vi "InitDrivebase.vi"   [LabVIEW 2020]
doc: "This VI initializes devices related directly to the drive subsystem."
uses:
  <vilib>/Rock Robotics/WPI/Solenoid/WPI_SolenoidChannel.ctl
  <vilib>/Rock Robotics/WPI/ThirdParty/Phoenix-LabVIEW/Motor Controller/Controls/CTRE_Phoenix_MotorControl_SupplyCurrentLimitConfiguration.ctl
  <vilib>/Rock Robotics/WPI/ThirdParty/Phoenix-LabVIEW/Motor Controller/Controls/CTRE_Phoenix_MotorControl_TalonFXInvertType.ctl
  <vilib>/Rock Robotics/WPI/ThirdParty/Phoenix-LabVIEW/Motor Controller/Controls/CTRE_Phoenix_MotorControl_NeutralMode.ctl
  <vilib>/Rock Robotics/WPI/ThirdParty/Phoenix-LabVIEW/Motor Controller/Controls/CTRE_Phoenix_MotorControl_FeedbackDevice_TalonFX.ctl
  <vilib>/Rock Robotics/WPI/ThirdParty/Phoenix-LabVIEW/Motor Controller/Controls/CTRE_Phoenix_MotorControl_StatusFrameEnhanced.ctl
  <vilib>/Rock Robotics/WPI/ThirdParty/Phoenix-LabVIEW/Motor Controller/Controls/CTRE_Phoenix_MotorControl_StatorCurrentLimitConfiguration.ctl
  <vilib>/Rock Robotics/WPI/Solenoid/WPI_SolenoidOpenDouble.vi
  GlobalDrivebase.vi
types:
  T1 = typedef "CTRE_Phoenix_MotorControl_StatorCurrentLimitConfiguration.ctl" = cluster{"Enable?":bool, "Current Limit":dbl, "Threshold Current":dbl, "Threshold Time":dbl}
  T2 = typedef "CTRE_Phoenix_MotorControl_StatusFrameEnhanced.ctl" = u16
  T3 = typedef "WPI_SolenoidChannel.ctl" = enum8{"Solenoid 0", "Solenoid 1", "Solenoid 2", "Solenoid 3", "Solenoid 4", "Solenoid 5", "Solenoid 6", "Solenoid 7", "Solenoid 8", "Solenoid 9", "Solenoid 10", "Solenoid 11", "Solenoid 12", "Solenoid 13", "Solenoid 14", "Solenoid 15", "Invalid"}
  T4 = typedef "CTRE_Phoenix_MotorControl_TalonFXInvertType.ctl" = enum16{"Counter-Clockwise", "Clockwise"}
  T5 = typedef "CTRE_Phoenix_MotorControl_FeedbackDevice_TalonFX.ctl" = i8
  T6 = typedef "CTRE_Phoenix_MotorControl_SupplyCurrentLimitConfiguration.ctl" = cluster{"Enable?":bool, "Current Limit":dbl, "Threshold Current":dbl, "Threshold Time":dbl}
  T7 = typedef "CTRE_Phoenix_MotorControl_NeutralMode.ctl" = enum8{"EEPROMSetting", "Override to Coast", "Override to Brake"}
  T8 = typedef "CTRE_PigeonIMU_DeviceRef.ctl" = cluster{"DeviceStatus":errorcluster, "Device Number":u8, "Type":T9, "Device ID":u32, "Handle":u64, "UsageFrame":u32, "Library Path":path}
  T9 = typedef "CTRE_PigeonIMU_ConnectionType.ctl" = u32
  T10 = typedef "WPI_MotorControlDeviceRef.ctl" = cluster{"DeviceStatus":errorcluster, "Type":T11, "PWM":cluster{"PWM Channel":T12, "DeadBand":T13}, "CAN":cluster{"Device Number":u8, "SetOutput VI Ref":variant, "GetOutput VI Ref":variant, "Enable VI Ref":variant, "Disable VI Ref":variant, "Data":variant}, "Invert":bool, "DIO PWM":cluster{"PWM \"Enable\" Channel":T12, "DIOChannel":T14, "PWM Rate":dbl}}
  T11 = typedef "WPI_MotorControlType.ctl" = enum16{"PWM", "CAN", "DIO PWM"}
  T12 = typedef "FPGA_DIOPWMChannel.ctl" = enum8{"PWM 0", "PWM 1", "PWM 2", "PWM 3", "PWM 4", "PWM 5", "PWM 6", "PWM 7", "PWM 8", "PWM 9", "PWM MXP 0", "PWM MXP 1", "PWM MXP 2", "PWM MXP 3", "PWM MXP 4", "PWM MXP 5", "PWM MXP 6", "PWM MXP 7", "PWM MXP 8", "PWM MXP 9", "Invalid"}
  T13 = typedef "WPI_PWMDeadband.ctl" = cluster{"Name":string, "maxPositivePwm":i32, "minPositivePwm":i32, "centerPwm":i32, "maxNegativePwm":i32, "minNegativePwm":i32, "angularRange":u16}
  T14 = typedef "FPGA_DIOChannel.ctl" = enum8{"DIO 0", "DIO 1", "DIO 2", "DIO 3", "DIO 4", "DIO 5", "DIO 6", "DIO 7", "DIO 8", "DIO 9", "DIO MXP 0", "DIO MXP 1", "DIO MXP 2", "DIO MXP 3", "DIO MXP 4", "DIO MXP 5", "DIO MXP 6", "DIO MXP 7", "DIO MXP 8", "DIO MXP 9", "DIO MXP 10", "DIO MXP 11", "DIO MXP 12", "DIO MXP 13", "DIO MXP 14", "DIO MXP 15", "SPI Port CS1", "SPI Port CS2", "SPI Port CS3", "SPI Port MISO", "SPI Port MOSI", "Invalid"}
  T15 = typedef "WPI_SolenoidDevRef.ctl" = cluster{"DevStatus":errorcluster, "Pneumatics Control Module":u8, "Forward Solenoid Channel":T3, "Reverse Solenoid Channel":T3}
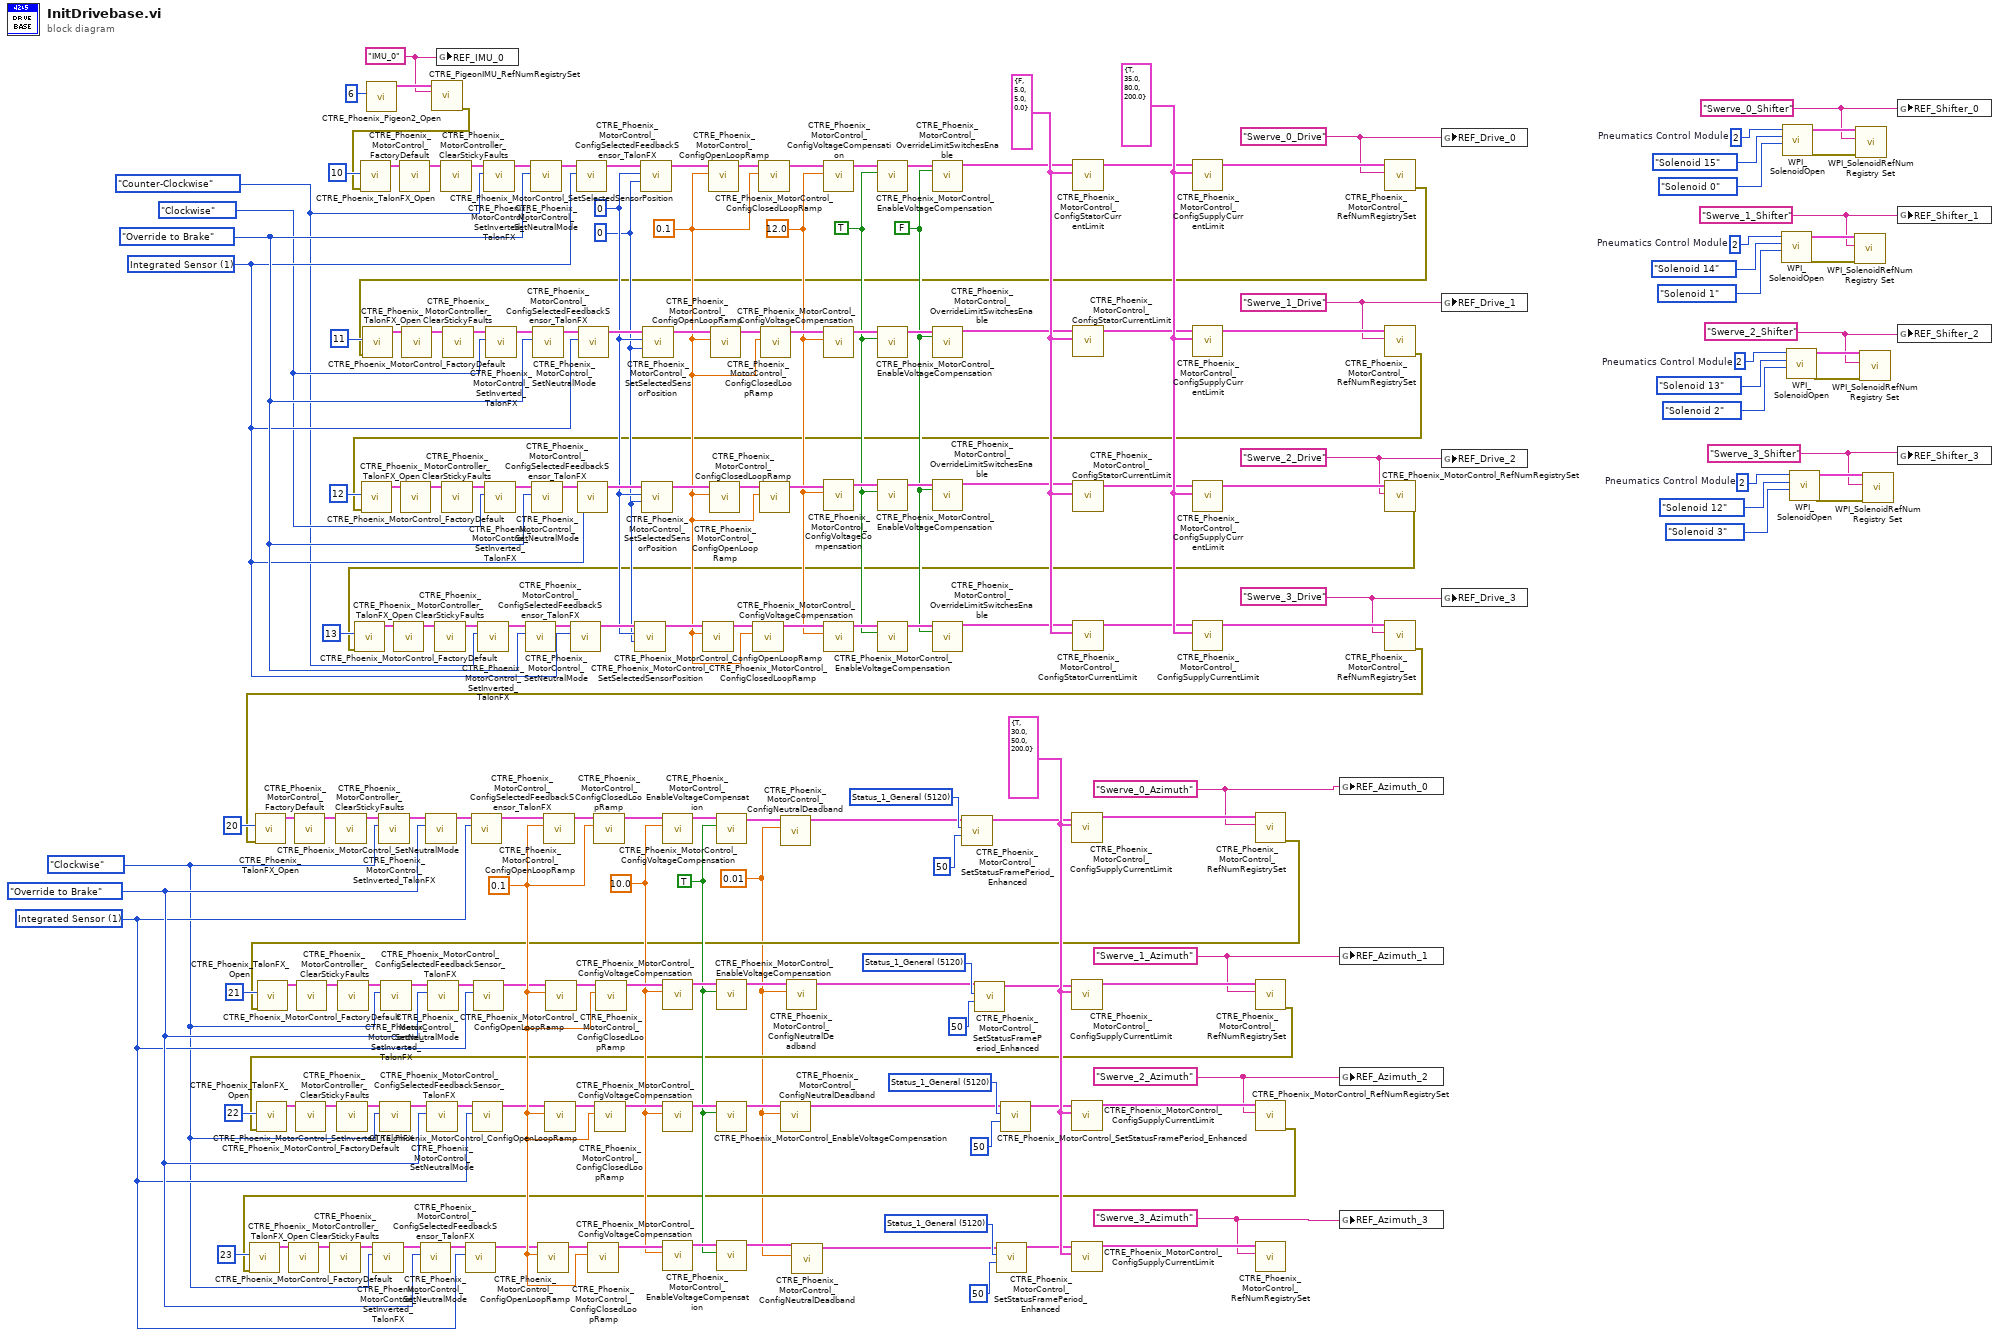
[diagram p0: block diagram]
diagram:
  w1 = "IMU_0" ("refnum name")
  w21 = 0.01 ("Percent Deadband")
  w34 = T1 {"Enable?"=FALSE, "Current Limit"=5.0, "Threshold Current"=5.0, "Threshold Time"=0.0} ("Stator Current Limit Configuration")
  w40 = T2 5120 items=["Status_1_General"=5120, "Status_2_Feedback0"=5184, "Status_3_Quadrature"=5248, "Status_4_AinTempVbat"=5312, "Status_6_Misc"=5440, "Status_7_CommStatus"=5504, "Status_8_PulseWidth"=5568, "Status_9_MotProfBuffer"=5632, "Status_10_MotionMagic"=5696, "Status_11_UartGadgeteer"=5760, "Status_12_Feedback1"=5824, "Status_13_Base_PIDF0"=5888, "Status_14_Turn_PIDF1"=5952, "Status_15_FirmwareApiStatus"=6016, "Status_Brushless_Current"=4672] ("Status Frame")
  w43 = T2 5120 items=["Status_1_General"=5120, "Status_2_Feedback0"=5184, "Status_3_Quadrature"=5248, "Status_4_AinTempVbat"=5312, "Status_6_Misc"=5440, "Status_7_CommStatus"=5504, "Status_8_PulseWidth"=5568, "Status_9_MotProfBuffer"=5632, "Status_10_MotionMagic"=5696, "Status_11_UartGadgeteer"=5760, "Status_12_Feedback1"=5824, "Status_13_Base_PIDF0"=5888, "Status_14_Turn_PIDF1"=5952, "Status_15_FirmwareApiStatus"=6016, "Status_Brushless_Current"=4672] ("Status Frame")
  w46 = T2 5120 items=["Status_1_General"=5120, "Status_2_Feedback0"=5184, "Status_3_Quadrature"=5248, "Status_4_AinTempVbat"=5312, "Status_6_Misc"=5440, "Status_7_CommStatus"=5504, "Status_8_PulseWidth"=5568, "Status_9_MotProfBuffer"=5632, "Status_10_MotionMagic"=5696, "Status_11_UartGadgeteer"=5760, "Status_12_Feedback1"=5824, "Status_13_Base_PIDF0"=5888, "Status_14_Turn_PIDF1"=5952, "Status_15_FirmwareApiStatus"=6016, "Status_Brushless_Current"=4672] ("Status Frame")
  w48 = T2 5120 items=["Status_1_General"=5120, "Status_2_Feedback0"=5184, "Status_3_Quadrature"=5248, "Status_4_AinTempVbat"=5312, "Status_6_Misc"=5440, "Status_7_CommStatus"=5504, "Status_8_PulseWidth"=5568, "Status_9_MotProfBuffer"=5632, "Status_10_MotionMagic"=5696, "Status_11_UartGadgeteer"=5760, "Status_12_Feedback1"=5824, "Status_13_Base_PIDF0"=5888, "Status_14_Turn_PIDF1"=5952, "Status_15_FirmwareApiStatus"=6016, "Status_Brushless_Current"=4672] ("Status Frame")
  w58 = FALSE ("Override Limit Switch Enable?")
  w13 = "Swerve_0_Shifter" ("refnum name")
  w68 = u8 2  # Pneumatics Control Module
  w12 = "Swerve_1_Shifter" ("refnum name")
  w73 = u8 2  # Pneumatics Control Module
  w11 = "Swerve_2_Shifter" ("refnum name")
  w78 = u8 2  # Pneumatics Control Module
  w79 = CTRE_Phoenix_MotorControl_TalonFXInvertType."Counter-Clockwise" ("Invert Type")
  w81 = TRUE ("Enable Voltage Compensation?")
  w82 = 10.0 ("Saturation Voltage")
  w83 = TRUE ("Enable Voltage Compensation?")
  w84 = 12.0 ("Saturation Voltage")
  w101 = T5 1 items=["Integrated Sensor"=1, "Sensor Sum (S0 + S1)"=9, "Sensor Difference (D0 - D1)"=10, "Remote Source 0"=11, "Remote Source 1"=12, "None"=14, "Software Emulated"=15] ("Talon FX Feedback Device")
  w104 = T6 {"Enable?"=TRUE, "Current Limit"=30.0, "Threshold Current"=50.0, "Threshold Time"=200.0} ("Supply Current Limit Configuration")
  w102 = 0.1 ("secondsFromNeutralToFull")
  w103 = CTRE_Phoenix_MotorControl_NeutralMode."Override to Brake" ("Motor Control Neutral Mode")
  w63 = CTRE_Phoenix_MotorControl_TalonFXInvertType."Clockwise" ("Invert Type")
  w5 = "Swerve_0_Azimuth" ("refnum name")
  w4 = "Swerve_1_Azimuth" ("refnum name")
  w3 = "Swerve_2_Azimuth" ("refnum name")
  w2 = "Swerve_3_Azimuth" ("refnum name")
  w140 = T5 1 items=["Integrated Sensor"=1, "Sensor Sum (S0 + S1)"=9, "Sensor Difference (D0 - D1)"=10, "Remote Source 0"=11, "Remote Source 1"=12, "None"=14, "Software Emulated"=15] ("Talon FX Feedback Device")
  w142 = T6 {"Enable?"=TRUE, "Current Limit"=35.0, "Threshold Current"=80.0, "Threshold Time"=200.0} ("Supply Current Limit Configuration")
  w137 = 0.1 ("secondsFromNeutralToFull")
  w138 = u32 0 ("pidLoopIdx")
  w139 = 0 ("New Sensor Position")
  w141 = CTRE_Phoenix_MotorControl_NeutralMode."Override to Brake" ("Motor Control Neutral Mode")
  w80 = CTRE_Phoenix_MotorControl_TalonFXInvertType."Clockwise" ("Invert Type")
  w9 = "Swerve_0_Drive" ("refnum name")
  w8 = "Swerve_1_Drive" ("refnum name")
  w7 = "Swerve_2_Drive" ("refnum name")
  w6 = "Swerve_3_Drive" ("refnum name")
  w10 = "Swerve_3_Shifter" ("refnum name")
  w187 = u8 2  # Pneumatics Control Module
  n1 = call <vilib>:"CTRE_Phoenix_Pigeon2_Open.vi"("Device Number"=u8 6) -> ("PigeonIMUDevRef"=w19:T8)  [unwired: 9 in, 1 out]
  n2 = call <vilib>:"CTRE_PigeonIMU_RefNumRegistrySet.vi"("refnum name"=w1, "PigeonIMUDevRef"=w19) -> ("error out"=w15:errorcluster)  [unwired: 8 in, 1 out]
  n3 = call <vilib>:"CTRE_Phoenix_TalonFX_Open.vi"("error in"=w15, "Device Number"=u8 10 ("Drive 4L")) -> ("PhoenixMotorControlDevRef"=w148:T10)  [unwired: 8 in, 1 out]
  n4 = call <vilib>:"CTRE_Phoenix_MotorControl_FactoryDefault.vi"("PhoenixMotorControlDevRef"=w148) -> ("PhoenixMotorControlDevRef"=w146:T10)  [unwired: 9 in, 1 out]
  n5 = global write "GlobalDrivebase.vi" "REF_IMU_0"(w1) -> ()
  n6 = call <vilib>:"CTRE_Phoenix_MotorController_ClearStickyFaults.vi"("PhoenixMotorControlDevRef"=w146) -> ("PhoenixMotorControlDevRef"=w145:T10)  [unwired: 9 in, 1 out]
  n7 = call <vilib>:"CTRE_Phoenix_MotorControl_SetInverted_TalonFX.vi"("Invert Type"=w79, "PhoenixMotorControlDevRef"=w145) -> ("PhoenixMotorControlDevRef"=w152:T10)  [unwired: 8 in, 1 out]
  n8 = call <vilib>:"CTRE_Phoenix_MotorControl_SetNeutralMode.vi"("Motor Control Neutral Mode"=w141, "PhoenixMotorControlDevRef"=w152) -> ("PhoenixMotorControlDevRef"=w144:T10)  [unwired: 8 in, 1 out]
  n9 = call <vilib>:"CTRE_Phoenix_MotorControl_ConfigSelectedFeedbackSensor_TalonFX.vi"("Talon FX Feedback Device"=w140, "PhoenixMotorControlDevRef"=w144) -> ("PhoenixMotorControlDevRef"=w143:T10)  [unwired: 8 in, 1 out]
  n10 = call <vilib>:"CTRE_Phoenix_MotorControl_SetSelectedSensorPosition.vi"("pidLoopIdx"=w138, "New Sensor Position"=w139, "PhoenixMotorControlDevRef"=w143) -> ("PhoenixMotorControlDevRef"=w151:T10)  [unwired: 7 in, 1 out]
  n11 = call <vilib>:"CTRE_Phoenix_MotorControl_ConfigOpenLoopRamp.vi"("secondsFromNeutralToFull"=w137, "PhoenixMotorControlDevRef"=w151) -> ("PhoenixMotorControlDevRef"=w147:T10)  [unwired: 8 in, 1 out]
  n12 = call <vilib>:"CTRE_Phoenix_MotorControl_ConfigClosedLoopRamp.vi"("secondsFromNeutralToFull"=w137, "PhoenixMotorControlDevRef"=w147) -> ("PhoenixMotorControlDevRef"=w92:T10)  [unwired: 8 in, 1 out]
  n13 = call <vilib>:"CTRE_Phoenix_MotorControl_ConfigVoltageCompensation.vi"("Saturation Voltage"=w84, "PhoenixMotorControlDevRef"=w92) -> ("PhoenixMotorControlDevRef"=w100:T10)  [unwired: 8 in, 1 out]
  n14 = call <vilib>:"CTRE_Phoenix_MotorControl_EnableVoltageCompensation.vi"("Enable Voltage Compensation?"=w83, "PhoenixMotorControlDevRef"=w100) -> ("PhoenixMotorControlDevRef"=w62:T10)  [unwired: 8 in, 1 out]
  n15 = call <vilib>:"CTRE_Phoenix_MotorControl_OverrideLimitSwitchesEnable.vi"("PhoenixMotorControlDevRef"=w62, "Override Limit Switch Enable?"=w58) -> ("PhoenixMotorControlDevRef"=w33:T10)  [unwired: 12 in, 1 out]
  n16 = call <vilib>:"CTRE_Phoenix_MotorControl_ConfigStatorCurrentLimit.vi"("Stator Current Limit Configuration"=w34, "PhoenixMotorControlDevRef"=w33) -> ("PhoenixMotorControlDevRef"=w38:T10)  [unwired: 8 in, 1 out]
  n17 = call <vilib>:"CTRE_Phoenix_MotorControl_ConfigSupplyCurrentLimit.vi"("Supply Current Limit Configuration"=w142, "PhoenixMotorControlDevRef"=w38) -> ("PhoenixMotorControlDevRef"=w150:T10)  [unwired: 8 in, 1 out]
  n18 = global write "GlobalDrivebase.vi" "REF_Azimuth_0"(w5) -> ()
  n19 = global write "GlobalDrivebase.vi" "REF_Azimuth_1"(w4) -> ()
  n20 = global write "GlobalDrivebase.vi" "REF_Azimuth_2"(w3) -> ()
  n21 = global write "GlobalDrivebase.vi" "REF_Azimuth_3"(w2) -> ()
  n22 = call <vilib>:"CTRE_Phoenix_MotorControl_RefNumRegistrySet.vi"("refnum name"=w9, "PhoenixMotorControlDevRef"=w150) -> ("error out"=w18:errorcluster)  [unwired: 8 in, 1 out]
  n23 = call <vilib>:"CTRE_Phoenix_TalonFX_Open.vi"("error in"=w18, "Device Number"=u8 11 ("Drive 4L")) -> ("PhoenixMotorControlDevRef"=w158:T10)  [unwired: 8 in, 1 out]
  n24 = call <vilib>:"CTRE_Phoenix_MotorControl_FactoryDefault.vi"("PhoenixMotorControlDevRef"=w158) -> ("PhoenixMotorControlDevRef"=w156:T10)  [unwired: 9 in, 1 out]
  n25 = call <vilib>:"CTRE_Phoenix_MotorController_ClearStickyFaults.vi"("PhoenixMotorControlDevRef"=w156) -> ("PhoenixMotorControlDevRef"=w155:T10)  [unwired: 9 in, 1 out]
  n26 = call <vilib>:"CTRE_Phoenix_MotorControl_SetInverted_TalonFX.vi"("Invert Type"=w80, "PhoenixMotorControlDevRef"=w155) -> ("PhoenixMotorControlDevRef"=w162:T10)  [unwired: 8 in, 1 out]
  n27 = call <vilib>:"CTRE_Phoenix_MotorControl_SetNeutralMode.vi"("Motor Control Neutral Mode"=w141, "PhoenixMotorControlDevRef"=w162) -> ("PhoenixMotorControlDevRef"=w154:T10)  [unwired: 8 in, 1 out]
  n28 = call <vilib>:"CTRE_Phoenix_MotorControl_ConfigSelectedFeedbackSensor_TalonFX.vi"("Talon FX Feedback Device"=w140, "PhoenixMotorControlDevRef"=w154) -> ("PhoenixMotorControlDevRef"=w153:T10)  [unwired: 8 in, 1 out]
  n29 = call <vilib>:"CTRE_Phoenix_MotorControl_SetSelectedSensorPosition.vi"("pidLoopIdx"=w138, "New Sensor Position"=w139, "PhoenixMotorControlDevRef"=w153) -> ("PhoenixMotorControlDevRef"=w161:T10)  [unwired: 7 in, 1 out]
  n30 = call <vilib>:"CTRE_Phoenix_MotorControl_ConfigOpenLoopRamp.vi"("secondsFromNeutralToFull"=w137, "PhoenixMotorControlDevRef"=w161) -> ("PhoenixMotorControlDevRef"=w157:T10)  [unwired: 8 in, 1 out]
  n31 = call <vilib>:"CTRE_Phoenix_MotorControl_ConfigClosedLoopRamp.vi"("secondsFromNeutralToFull"=w137, "PhoenixMotorControlDevRef"=w157) -> ("PhoenixMotorControlDevRef"=w91:T10)  [unwired: 8 in, 1 out]
  n32 = call <vilib>:"CTRE_Phoenix_MotorControl_ConfigVoltageCompensation.vi"("Saturation Voltage"=w84, "PhoenixMotorControlDevRef"=w91) -> ("PhoenixMotorControlDevRef"=w99:T10)  [unwired: 8 in, 1 out]
  n33 = call <vilib>:"CTRE_Phoenix_MotorControl_EnableVoltageCompensation.vi"("Enable Voltage Compensation?"=w83, "PhoenixMotorControlDevRef"=w99) -> ("PhoenixMotorControlDevRef"=w61:T10)  [unwired: 8 in, 1 out]
  n34 = call <vilib>:"CTRE_Phoenix_MotorControl_OverrideLimitSwitchesEnable.vi"("PhoenixMotorControlDevRef"=w61, "Override Limit Switch Enable?"=w58) -> ("PhoenixMotorControlDevRef"=w32:T10)  [unwired: 12 in, 1 out]
  n35 = call <vilib>:"CTRE_Phoenix_MotorControl_ConfigStatorCurrentLimit.vi"("Stator Current Limit Configuration"=w34, "PhoenixMotorControlDevRef"=w32) -> ("PhoenixMotorControlDevRef"=w37:T10)  [unwired: 8 in, 1 out]
  n36 = call <vilib>:"CTRE_Phoenix_MotorControl_ConfigSupplyCurrentLimit.vi"("Supply Current Limit Configuration"=w142, "PhoenixMotorControlDevRef"=w37) -> ("PhoenixMotorControlDevRef"=w160:T10)  [unwired: 8 in, 1 out]
  n37 = call <vilib>:"CTRE_Phoenix_MotorControl_RefNumRegistrySet.vi"("refnum name"=w8, "PhoenixMotorControlDevRef"=w160) -> ("error out"=w17:errorcluster)  [unwired: 8 in, 1 out]
  n38 = call <vilib>:"CTRE_Phoenix_TalonFX_Open.vi"("error in"=w17, "Device Number"=u8 12 ("Drive 4L")) -> ("PhoenixMotorControlDevRef"=w168:T10)  [unwired: 8 in, 1 out]
  n39 = call <vilib>:"CTRE_Phoenix_MotorControl_FactoryDefault.vi"("PhoenixMotorControlDevRef"=w168) -> ("PhoenixMotorControlDevRef"=w166:T10)  [unwired: 9 in, 1 out]
  n40 = call <vilib>:"CTRE_Phoenix_MotorController_ClearStickyFaults.vi"("PhoenixMotorControlDevRef"=w166) -> ("PhoenixMotorControlDevRef"=w165:T10)  [unwired: 9 in, 1 out]
  n41 = call <vilib>:"CTRE_Phoenix_MotorControl_SetInverted_TalonFX.vi"("Invert Type"=w80, "PhoenixMotorControlDevRef"=w165) -> ("PhoenixMotorControlDevRef"=w172:T10)  [unwired: 8 in, 1 out]
  n42 = call <vilib>:"CTRE_Phoenix_MotorControl_SetNeutralMode.vi"("Motor Control Neutral Mode"=w141, "PhoenixMotorControlDevRef"=w172) -> ("PhoenixMotorControlDevRef"=w164:T10)  [unwired: 8 in, 1 out]
  n43 = call <vilib>:"CTRE_Phoenix_MotorControl_ConfigSelectedFeedbackSensor_TalonFX.vi"("Talon FX Feedback Device"=w140, "PhoenixMotorControlDevRef"=w164) -> ("PhoenixMotorControlDevRef"=w163:T10)  [unwired: 8 in, 1 out]
  n44 = call <vilib>:"CTRE_Phoenix_MotorControl_SetSelectedSensorPosition.vi"("pidLoopIdx"=w138, "New Sensor Position"=w139, "PhoenixMotorControlDevRef"=w163) -> ("PhoenixMotorControlDevRef"=w171:T10)  [unwired: 7 in, 1 out]
  n45 = call <vilib>:"CTRE_Phoenix_MotorControl_ConfigOpenLoopRamp.vi"("secondsFromNeutralToFull"=w137, "PhoenixMotorControlDevRef"=w171) -> ("PhoenixMotorControlDevRef"=w167:T10)  [unwired: 8 in, 1 out]
  n46 = call <vilib>:"CTRE_Phoenix_MotorControl_ConfigClosedLoopRamp.vi"("secondsFromNeutralToFull"=w137, "PhoenixMotorControlDevRef"=w167) -> ("PhoenixMotorControlDevRef"=w90:T10)  [unwired: 8 in, 1 out]
  n47 = call <vilib>:"CTRE_Phoenix_MotorControl_ConfigVoltageCompensation.vi"("Saturation Voltage"=w84, "PhoenixMotorControlDevRef"=w90) -> ("PhoenixMotorControlDevRef"=w98:T10)  [unwired: 8 in, 1 out]
  n48 = call <vilib>:"CTRE_Phoenix_MotorControl_EnableVoltageCompensation.vi"("Enable Voltage Compensation?"=w83, "PhoenixMotorControlDevRef"=w98) -> ("PhoenixMotorControlDevRef"=w60:T10)  [unwired: 8 in, 1 out]
  n49 = call <vilib>:"CTRE_Phoenix_MotorControl_OverrideLimitSwitchesEnable.vi"("PhoenixMotorControlDevRef"=w60, "Override Limit Switch Enable?"=w58) -> ("PhoenixMotorControlDevRef"=w31:T10)  [unwired: 12 in, 1 out]
  n50 = call <vilib>:"CTRE_Phoenix_MotorControl_ConfigStatorCurrentLimit.vi"("Stator Current Limit Configuration"=w34, "PhoenixMotorControlDevRef"=w31) -> ("PhoenixMotorControlDevRef"=w36:T10)  [unwired: 8 in, 1 out]
  n51 = call <vilib>:"CTRE_Phoenix_MotorControl_ConfigSupplyCurrentLimit.vi"("Supply Current Limit Configuration"=w142, "PhoenixMotorControlDevRef"=w36) -> ("PhoenixMotorControlDevRef"=w170:T10)  [unwired: 8 in, 1 out]
  n52 = call <vilib>:"CTRE_Phoenix_MotorControl_RefNumRegistrySet.vi"("refnum name"=w7, "PhoenixMotorControlDevRef"=w170) -> ("error out"=w16:errorcluster)  [unwired: 8 in, 1 out]
  n53 = call <vilib>:"CTRE_Phoenix_TalonFX_Open.vi"("error in"=w16, "Device Number"=u8 13 ("Drive 4L")) -> ("PhoenixMotorControlDevRef"=w178:T10)  [unwired: 8 in, 1 out]
  n54 = call <vilib>:"CTRE_Phoenix_MotorControl_FactoryDefault.vi"("PhoenixMotorControlDevRef"=w178) -> ("PhoenixMotorControlDevRef"=w176:T10)  [unwired: 9 in, 1 out]
  n55 = call <vilib>:"CTRE_Phoenix_MotorController_ClearStickyFaults.vi"("PhoenixMotorControlDevRef"=w176) -> ("PhoenixMotorControlDevRef"=w175:T10)  [unwired: 9 in, 1 out]
  n56 = call <vilib>:"CTRE_Phoenix_MotorControl_SetInverted_TalonFX.vi"("Invert Type"=w79, "PhoenixMotorControlDevRef"=w175) -> ("PhoenixMotorControlDevRef"=w182:T10)  [unwired: 8 in, 1 out]
  n57 = call <vilib>:"CTRE_Phoenix_MotorControl_SetNeutralMode.vi"("Motor Control Neutral Mode"=w141, "PhoenixMotorControlDevRef"=w182) -> ("PhoenixMotorControlDevRef"=w174:T10)  [unwired: 8 in, 1 out]
  n58 = call <vilib>:"CTRE_Phoenix_MotorControl_ConfigSelectedFeedbackSensor_TalonFX.vi"("Talon FX Feedback Device"=w140, "PhoenixMotorControlDevRef"=w174) -> ("PhoenixMotorControlDevRef"=w173:T10)  [unwired: 8 in, 1 out]
  n59 = call <vilib>:"CTRE_Phoenix_MotorControl_SetSelectedSensorPosition.vi"("pidLoopIdx"=w138, "New Sensor Position"=w139, "PhoenixMotorControlDevRef"=w173) -> ("PhoenixMotorControlDevRef"=w181:T10)  [unwired: 7 in, 1 out]
  n60 = call <vilib>:"CTRE_Phoenix_MotorControl_ConfigOpenLoopRamp.vi"("secondsFromNeutralToFull"=w137, "PhoenixMotorControlDevRef"=w181) -> ("PhoenixMotorControlDevRef"=w177:T10)  [unwired: 8 in, 1 out]
  n61 = call <vilib>:"CTRE_Phoenix_MotorControl_ConfigClosedLoopRamp.vi"("secondsFromNeutralToFull"=w137, "PhoenixMotorControlDevRef"=w177) -> ("PhoenixMotorControlDevRef"=w89:T10)  [unwired: 8 in, 1 out]
  n62 = call <vilib>:"CTRE_Phoenix_MotorControl_ConfigVoltageCompensation.vi"("Saturation Voltage"=w84, "PhoenixMotorControlDevRef"=w89) -> ("PhoenixMotorControlDevRef"=w97:T10)  [unwired: 8 in, 1 out]
  n63 = call <vilib>:"CTRE_Phoenix_MotorControl_EnableVoltageCompensation.vi"("Enable Voltage Compensation?"=w83, "PhoenixMotorControlDevRef"=w97) -> ("PhoenixMotorControlDevRef"=w59:T10)  [unwired: 8 in, 1 out]
  n64 = call <vilib>:"CTRE_Phoenix_MotorControl_OverrideLimitSwitchesEnable.vi"("PhoenixMotorControlDevRef"=w59, "Override Limit Switch Enable?"=w58) -> ("PhoenixMotorControlDevRef"=w30:T10)  [unwired: 12 in, 1 out]
  n65 = call <vilib>:"CTRE_Phoenix_MotorControl_ConfigStatorCurrentLimit.vi"("Stator Current Limit Configuration"=w34, "PhoenixMotorControlDevRef"=w30) -> ("PhoenixMotorControlDevRef"=w35:T10)  [unwired: 8 in, 1 out]
  n66 = call <vilib>:"CTRE_Phoenix_MotorControl_ConfigSupplyCurrentLimit.vi"("Supply Current Limit Configuration"=w142, "PhoenixMotorControlDevRef"=w35) -> ("PhoenixMotorControlDevRef"=w180:T10)  [unwired: 8 in, 1 out]
  n67 = call <vilib>:"CTRE_Phoenix_MotorControl_RefNumRegistrySet.vi"("refnum name"=w6, "PhoenixMotorControlDevRef"=w180) -> ("error out"=w14:errorcluster)  [unwired: 8 in, 1 out]
  n68 = call <vilib>:"CTRE_Phoenix_TalonFX_Open.vi"("error in"=w14, "Device Number"=u8 20 ("Drive 4L")) -> ("PhoenixMotorControlDevRef"=w109:T10)  [unwired: 8 in, 1 out]
  n69 = call <vilib>:"CTRE_Phoenix_MotorControl_FactoryDefault.vi"("PhoenixMotorControlDevRef"=w109) -> ("PhoenixMotorControlDevRef"=w107:T10)  [unwired: 9 in, 1 out]
  n70 = call <vilib>:"CTRE_Phoenix_MotorController_ClearStickyFaults.vi"("PhoenixMotorControlDevRef"=w107) -> ("PhoenixMotorControlDevRef"=w106:T10)  [unwired: 9 in, 1 out]
  n71 = call <vilib>:"CTRE_Phoenix_MotorControl_SetInverted_TalonFX.vi"("Invert Type"=w63, "PhoenixMotorControlDevRef"=w106) -> ("PhoenixMotorControlDevRef"=w112:T10)  [unwired: 8 in, 1 out]
  n72 = call <vilib>:"CTRE_Phoenix_MotorControl_SetNeutralMode.vi"("Motor Control Neutral Mode"=w103, "PhoenixMotorControlDevRef"=w112) -> ("PhoenixMotorControlDevRef"=w105:T10)  [unwired: 8 in, 1 out]
  n73 = call <vilib>:"CTRE_Phoenix_MotorControl_ConfigSelectedFeedbackSensor_TalonFX.vi"("Talon FX Feedback Device"=w101, "PhoenixMotorControlDevRef"=w105) -> ("PhoenixMotorControlDevRef"=w54:T10)  [unwired: 8 in, 1 out]
  n74 = call <vilib>:"CTRE_Phoenix_MotorControl_ConfigOpenLoopRamp.vi"("secondsFromNeutralToFull"=w102, "PhoenixMotorControlDevRef"=w54) -> ("PhoenixMotorControlDevRef"=w108:T10)  [unwired: 8 in, 1 out]
  n75 = call <vilib>:"CTRE_Phoenix_MotorControl_ConfigClosedLoopRamp.vi"("secondsFromNeutralToFull"=w102, "PhoenixMotorControlDevRef"=w108) -> ("PhoenixMotorControlDevRef"=w88:T10)  [unwired: 8 in, 1 out]
  n76 = call <vilib>:"CTRE_Phoenix_MotorControl_ConfigVoltageCompensation.vi"("Saturation Voltage"=w82, "PhoenixMotorControlDevRef"=w88) -> ("PhoenixMotorControlDevRef"=w96:T10)  [unwired: 8 in, 1 out]
  n77 = call <vilib>:"CTRE_Phoenix_MotorControl_EnableVoltageCompensation.vi"("Enable Voltage Compensation?"=w81, "PhoenixMotorControlDevRef"=w96) -> ("PhoenixMotorControlDevRef"=w29:T10)  [unwired: 8 in, 1 out]
  n78 = call <vilib>:"CTRE_Phoenix_MotorControl_ConfigNeutralDeadband.vi"("Percent Deadband"=w21, "PhoenixMotorControlDevRef"=w29) -> ("PhoenixMotorControlDevRef"=w28:T10)  [unwired: 8 in, 1 out]
  n79 = call <vilib>:"CTRE_Phoenix_MotorControl_SetStatusFramePeriod_Enhanced.vi"("periodMs"=50, "Status Frame"=w48, "PhoenixMotorControlDevRef"=w28) -> ("PhoenixMotorControlDevRef"=w49:T10)  [unwired: 7 in, 1 out]
  n80 = call <vilib>:"CTRE_Phoenix_MotorControl_ConfigSupplyCurrentLimit.vi"("Supply Current Limit Configuration"=w104, "PhoenixMotorControlDevRef"=w49) -> ("PhoenixMotorControlDevRef"=w111:T10)  [unwired: 8 in, 1 out]
  n81 = call <vilib>:"CTRE_Phoenix_MotorControl_RefNumRegistrySet.vi"("refnum name"=w5, "PhoenixMotorControlDevRef"=w111) -> ("error out"=w53:errorcluster)  [unwired: 8 in, 1 out]
  n82 = call <vilib>:"CTRE_Phoenix_TalonFX_Open.vi"("error in"=w53, "Device Number"=u8 21 ("Drive 4L")) -> ("PhoenixMotorControlDevRef"=w117:T10)  [unwired: 8 in, 1 out]
  n83 = call <vilib>:"CTRE_Phoenix_MotorControl_FactoryDefault.vi"("PhoenixMotorControlDevRef"=w117) -> ("PhoenixMotorControlDevRef"=w115:T10)  [unwired: 9 in, 1 out]
  n84 = call <vilib>:"CTRE_Phoenix_MotorController_ClearStickyFaults.vi"("PhoenixMotorControlDevRef"=w115) -> ("PhoenixMotorControlDevRef"=w114:T10)  [unwired: 9 in, 1 out]
  n85 = call <vilib>:"CTRE_Phoenix_MotorControl_SetInverted_TalonFX.vi"("Invert Type"=w63, "PhoenixMotorControlDevRef"=w114) -> ("PhoenixMotorControlDevRef"=w120:T10)  [unwired: 8 in, 1 out]
  n86 = call <vilib>:"CTRE_Phoenix_MotorControl_SetNeutralMode.vi"("Motor Control Neutral Mode"=w103, "PhoenixMotorControlDevRef"=w120) -> ("PhoenixMotorControlDevRef"=w113:T10)  [unwired: 8 in, 1 out]
  n87 = call <vilib>:"CTRE_Phoenix_MotorControl_ConfigSelectedFeedbackSensor_TalonFX.vi"("Talon FX Feedback Device"=w101, "PhoenixMotorControlDevRef"=w113) -> ("PhoenixMotorControlDevRef"=w55:T10)  [unwired: 8 in, 1 out]
  n88 = call <vilib>:"CTRE_Phoenix_MotorControl_ConfigOpenLoopRamp.vi"("secondsFromNeutralToFull"=w102, "PhoenixMotorControlDevRef"=w55) -> ("PhoenixMotorControlDevRef"=w116:T10)  [unwired: 8 in, 1 out]
  n89 = call <vilib>:"CTRE_Phoenix_MotorControl_ConfigClosedLoopRamp.vi"("secondsFromNeutralToFull"=w102, "PhoenixMotorControlDevRef"=w116) -> ("PhoenixMotorControlDevRef"=w87:T10)  [unwired: 8 in, 1 out]
  n90 = call <vilib>:"CTRE_Phoenix_MotorControl_ConfigVoltageCompensation.vi"("Saturation Voltage"=w82, "PhoenixMotorControlDevRef"=w87) -> ("PhoenixMotorControlDevRef"=w95:T10)  [unwired: 8 in, 1 out]
  n91 = call <vilib>:"CTRE_Phoenix_MotorControl_EnableVoltageCompensation.vi"("Enable Voltage Compensation?"=w81, "PhoenixMotorControlDevRef"=w95) -> ("PhoenixMotorControlDevRef"=w27:T10)  [unwired: 8 in, 1 out]
  n92 = call <vilib>:"CTRE_Phoenix_MotorControl_ConfigNeutralDeadband.vi"("Percent Deadband"=w21, "PhoenixMotorControlDevRef"=w27) -> ("PhoenixMotorControlDevRef"=w26:T10)  [unwired: 8 in, 1 out]
  n93 = call <vilib>:"CTRE_Phoenix_MotorControl_SetStatusFramePeriod_Enhanced.vi"("periodMs"=50, "Status Frame"=w46, "PhoenixMotorControlDevRef"=w26) -> ("PhoenixMotorControlDevRef"=w45:T10)  [unwired: 7 in, 1 out]
  n94 = call <vilib>:"CTRE_Phoenix_MotorControl_ConfigSupplyCurrentLimit.vi"("Supply Current Limit Configuration"=w104, "PhoenixMotorControlDevRef"=w45) -> ("PhoenixMotorControlDevRef"=w119:T10)  [unwired: 8 in, 1 out]
  n95 = call <vilib>:"CTRE_Phoenix_MotorControl_RefNumRegistrySet.vi"("refnum name"=w4, "PhoenixMotorControlDevRef"=w119) -> ("error out"=w52:errorcluster)  [unwired: 8 in, 1 out]
  n96 = call <vilib>:"CTRE_Phoenix_TalonFX_Open.vi"("error in"=w52, "Device Number"=u8 22 ("Drive 4L")) -> ("PhoenixMotorControlDevRef"=w125:T10)  [unwired: 8 in, 1 out]
  n97 = call <vilib>:"CTRE_Phoenix_MotorControl_FactoryDefault.vi"("PhoenixMotorControlDevRef"=w125) -> ("PhoenixMotorControlDevRef"=w123:T10)  [unwired: 9 in, 1 out]
  n98 = call <vilib>:"CTRE_Phoenix_MotorController_ClearStickyFaults.vi"("PhoenixMotorControlDevRef"=w123) -> ("PhoenixMotorControlDevRef"=w122:T10)  [unwired: 9 in, 1 out]
  n99 = call <vilib>:"CTRE_Phoenix_MotorControl_SetInverted_TalonFX.vi"("Invert Type"=w63, "PhoenixMotorControlDevRef"=w122) -> ("PhoenixMotorControlDevRef"=w128:T10)  [unwired: 8 in, 1 out]
  n100 = call <vilib>:"CTRE_Phoenix_MotorControl_SetNeutralMode.vi"("Motor Control Neutral Mode"=w103, "PhoenixMotorControlDevRef"=w128) -> ("PhoenixMotorControlDevRef"=w121:T10)  [unwired: 8 in, 1 out]
  n101 = call <vilib>:"CTRE_Phoenix_MotorControl_ConfigSelectedFeedbackSensor_TalonFX.vi"("Talon FX Feedback Device"=w101, "PhoenixMotorControlDevRef"=w121) -> ("PhoenixMotorControlDevRef"=w56:T10)  [unwired: 8 in, 1 out]
  n102 = call <vilib>:"CTRE_Phoenix_MotorControl_ConfigOpenLoopRamp.vi"("secondsFromNeutralToFull"=w102, "PhoenixMotorControlDevRef"=w56) -> ("PhoenixMotorControlDevRef"=w124:T10)  [unwired: 8 in, 1 out]
  n103 = call <vilib>:"CTRE_Phoenix_MotorControl_ConfigClosedLoopRamp.vi"("secondsFromNeutralToFull"=w102, "PhoenixMotorControlDevRef"=w124) -> ("PhoenixMotorControlDevRef"=w86:T10)  [unwired: 8 in, 1 out]
  n104 = call <vilib>:"CTRE_Phoenix_MotorControl_ConfigVoltageCompensation.vi"("Saturation Voltage"=w82, "PhoenixMotorControlDevRef"=w86) -> ("PhoenixMotorControlDevRef"=w94:T10)  [unwired: 8 in, 1 out]
  n105 = call <vilib>:"CTRE_Phoenix_MotorControl_EnableVoltageCompensation.vi"("Enable Voltage Compensation?"=w81, "PhoenixMotorControlDevRef"=w94) -> ("PhoenixMotorControlDevRef"=w25:T10)  [unwired: 8 in, 1 out]
  n106 = call <vilib>:"CTRE_Phoenix_MotorControl_ConfigNeutralDeadband.vi"("Percent Deadband"=w21, "PhoenixMotorControlDevRef"=w25) -> ("PhoenixMotorControlDevRef"=w24:T10)  [unwired: 8 in, 1 out]
  n107 = call <vilib>:"CTRE_Phoenix_MotorControl_SetStatusFramePeriod_Enhanced.vi"("periodMs"=50, "Status Frame"=w43, "PhoenixMotorControlDevRef"=w24) -> ("PhoenixMotorControlDevRef"=w42:T10)  [unwired: 7 in, 1 out]
  n108 = call <vilib>:"CTRE_Phoenix_MotorControl_ConfigSupplyCurrentLimit.vi"("Supply Current Limit Configuration"=w104, "PhoenixMotorControlDevRef"=w42) -> ("PhoenixMotorControlDevRef"=w127:T10)  [unwired: 8 in, 1 out]
  n109 = call <vilib>:"CTRE_Phoenix_MotorControl_RefNumRegistrySet.vi"("refnum name"=w3, "PhoenixMotorControlDevRef"=w127) -> ("error out"=w51:errorcluster)  [unwired: 8 in, 1 out]
  n110 = call <vilib>:"CTRE_Phoenix_TalonFX_Open.vi"("error in"=w51, "Device Number"=u8 23 ("Drive 4L")) -> ("PhoenixMotorControlDevRef"=w133:T10)  [unwired: 8 in, 1 out]
  n111 = call <vilib>:"CTRE_Phoenix_MotorControl_FactoryDefault.vi"("PhoenixMotorControlDevRef"=w133) -> ("PhoenixMotorControlDevRef"=w131:T10)  [unwired: 9 in, 1 out]
  n112 = call <vilib>:"CTRE_Phoenix_MotorController_ClearStickyFaults.vi"("PhoenixMotorControlDevRef"=w131) -> ("PhoenixMotorControlDevRef"=w130:T10)  [unwired: 9 in, 1 out]
  n113 = call <vilib>:"CTRE_Phoenix_MotorControl_SetInverted_TalonFX.vi"("Invert Type"=w63, "PhoenixMotorControlDevRef"=w130) -> ("PhoenixMotorControlDevRef"=w136:T10)  [unwired: 8 in, 1 out]
  n114 = call <vilib>:"CTRE_Phoenix_MotorControl_SetNeutralMode.vi"("Motor Control Neutral Mode"=w103, "PhoenixMotorControlDevRef"=w136) -> ("PhoenixMotorControlDevRef"=w129:T10)  [unwired: 8 in, 1 out]
  n115 = call <vilib>:"CTRE_Phoenix_MotorControl_ConfigSelectedFeedbackSensor_TalonFX.vi"("Talon FX Feedback Device"=w101, "PhoenixMotorControlDevRef"=w129) -> ("PhoenixMotorControlDevRef"=w57:T10)  [unwired: 8 in, 1 out]
  n116 = call <vilib>:"CTRE_Phoenix_MotorControl_ConfigOpenLoopRamp.vi"("secondsFromNeutralToFull"=w102, "PhoenixMotorControlDevRef"=w57) -> ("PhoenixMotorControlDevRef"=w132:T10)  [unwired: 8 in, 1 out]
  n117 = call <vilib>:"CTRE_Phoenix_MotorControl_ConfigClosedLoopRamp.vi"("secondsFromNeutralToFull"=w102, "PhoenixMotorControlDevRef"=w132) -> ("PhoenixMotorControlDevRef"=w85:T10)  [unwired: 8 in, 1 out]
  n118 = call <vilib>:"CTRE_Phoenix_MotorControl_ConfigVoltageCompensation.vi"("Saturation Voltage"=w82, "PhoenixMotorControlDevRef"=w85) -> ("PhoenixMotorControlDevRef"=w93:T10)  [unwired: 8 in, 1 out]
  n119 = call <vilib>:"CTRE_Phoenix_MotorControl_EnableVoltageCompensation.vi"("Enable Voltage Compensation?"=w81, "PhoenixMotorControlDevRef"=w93) -> ("PhoenixMotorControlDevRef"=w23:T10)  [unwired: 8 in, 1 out]
  n120 = call <vilib>:"CTRE_Phoenix_MotorControl_ConfigNeutralDeadband.vi"("Percent Deadband"=w21, "PhoenixMotorControlDevRef"=w23) -> ("PhoenixMotorControlDevRef"=w22:T10)  [unwired: 8 in, 1 out]
  n121 = call <vilib>:"CTRE_Phoenix_MotorControl_SetStatusFramePeriod_Enhanced.vi"("periodMs"=50, "Status Frame"=w40, "PhoenixMotorControlDevRef"=w22) -> ("PhoenixMotorControlDevRef"=w39:T10)  [unwired: 7 in, 1 out]
  n122 = call <vilib>:"CTRE_Phoenix_MotorControl_ConfigSupplyCurrentLimit.vi"("Supply Current Limit Configuration"=w104, "PhoenixMotorControlDevRef"=w39) -> ("PhoenixMotorControlDevRef"=w135:T10)  [unwired: 8 in, 1 out]
  n123 = call <vilib>:"CTRE_Phoenix_MotorControl_RefNumRegistrySet.vi"("refnum name"=w2, "PhoenixMotorControlDevRef"=w135) -> ()  [unwired: 8 in, 2 out]
  n124 = global write "GlobalDrivebase.vi" "REF_Drive_0"(w9) -> ()
  n125 = global write "GlobalDrivebase.vi" "REF_Drive_1"(w8) -> ()
  n126 = global write "GlobalDrivebase.vi" "REF_Drive_2"(w7) -> ()
  n127 = global write "GlobalDrivebase.vi" "REF_Drive_3"(w6) -> ()
  n128 = call-poly <vilib>:"WPI_SolenoidOpen.vi"("Reverse Solenoid Channel"=WPI_SolenoidChannel."Solenoid 1", "Forward Solenoid Channel"=WPI_SolenoidChannel."Solenoid 14", "Pneumatics Device (def)"=w73) -> ("error out"=w69:errorcluster, "SolenoidDevRef"=w70:T15)  [unwired: 7 in]
  n129 = call-poly <vilib>:"WPI_SolenoidOpen.vi"("Reverse Solenoid Channel"=WPI_SolenoidChannel."Solenoid 0", "Forward Solenoid Channel"=WPI_SolenoidChannel."Solenoid 15", "Pneumatics Device (def)"=w68) -> ("error out"=w64:errorcluster, "SolenoidDevRef"=w65:T15)  [unwired: 7 in]
  n130 = call-poly <vilib>:"WPI_SolenoidOpen.vi"("Reverse Solenoid Channel"=WPI_SolenoidChannel."Solenoid 2", "Forward Solenoid Channel"=WPI_SolenoidChannel."Solenoid 13", "Pneumatics Device (def)"=w78) -> ("error out"=w74:errorcluster, "SolenoidDevRef"=w75:T15)  [unwired: 7 in]
  n131 = call-poly <vilib>:"WPI_SolenoidOpen.vi"("Reverse Solenoid Channel"=WPI_SolenoidChannel."Solenoid 3", "Forward Solenoid Channel"=WPI_SolenoidChannel."Solenoid 12", "Pneumatics Device (def)"=w187) -> ("error out"=w183:errorcluster, "SolenoidDevRef"=w184:T15)  [unwired: 7 in]
  n132 = call <vilib>:"WPI_SolenoidRefNum Registry Set.vi"("error in (no error)"=w69, "refnum name"=w12, "SolenoidDevRef"=w70) -> ()  [unwired: 7 in, 2 out]
  n133 = call <vilib>:"WPI_SolenoidRefNum Registry Set.vi"("error in (no error)"=w64, "refnum name"=w13, "SolenoidDevRef"=w65) -> ()  [unwired: 7 in, 2 out]
  n134 = call <vilib>:"WPI_SolenoidRefNum Registry Set.vi"("error in (no error)"=w74, "refnum name"=w11, "SolenoidDevRef"=w75) -> ()  [unwired: 7 in, 2 out]
  n135 = call <vilib>:"WPI_SolenoidRefNum Registry Set.vi"("error in (no error)"=w183, "refnum name"=w10, "SolenoidDevRef"=w184) -> ()  [unwired: 7 in, 2 out]
  n136 = global write "GlobalDrivebase.vi" "REF_Shifter_0"(w13) -> ()
  n137 = global write "GlobalDrivebase.vi" "REF_Shifter_1"(w12) -> ()
  n138 = global write "GlobalDrivebase.vi" "REF_Shifter_2"(w11) -> ()
  n139 = global write "GlobalDrivebase.vi" "REF_Shifter_3"(w10) -> ()
